vi "Stop apt.vi"(8 "error in (no error)":errorcluster, 11 "Hardware Resources In":T1={"Piezo Serial Number"=41848555, "MG17Piezo"=refnum, "Setpoint (um)"=0.0}) -> (0 "error out":errorcluster)   [LabVIEW 2013, in "Piezo.lvlib"]
uses:
  Piezo.lvlib
  Hardware Configuration.ctl
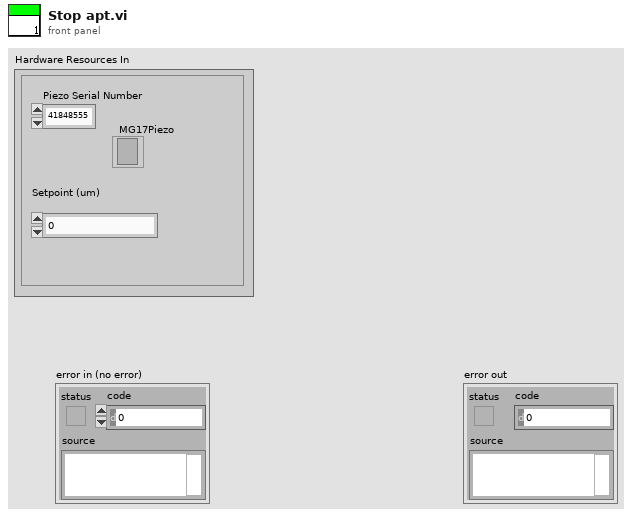
[diagram p1: front panel]
types:
  T1 = typedef "Piezo.lvlib/Hardware Configuration.ctl" = cluster{"Piezo Serial Number":i32, "MG17Piezo":refnum<k7>, "Setpoint (um)":sgl}
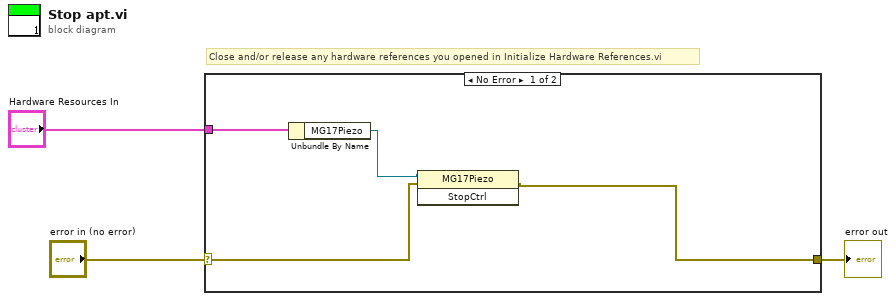
[diagram p0: block diagram]
diagram:
  # "Close and/or release any hardware references you opened in Initialize Hardware References.vi"
  n1 = case shown="No Error" "error in (no error)" {
    selector: "error in (no error)" -> [w5 w8]
    tunnel: [w4 w8] -> w2
    tunnel: "Hardware Resources In" -> [w7 _]
    frame No Error {
      n2 = Unbundle By Name(w7) -> ("MG17Piezo"=w6:refnum<k7>)
      n3 = invoke class="MG17Piezo" method="StopCtrl"(reference=w6, error in=w5) -> (error out=w4:errorcluster)  [unwired: 1 in, 2 out]
    }
    frame Error {
    }
  }
  "error out" <- w2
